vi "SmallestAngle.vi"(10 "Angle 2":dbl, 11 "Angle 1":dbl) -> (3 "Smallest Difference":dbl)   [LabVIEW 2016]
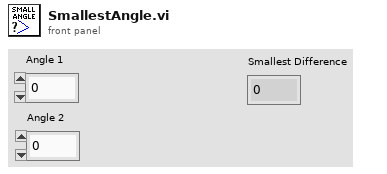
[diagram p1: front panel]
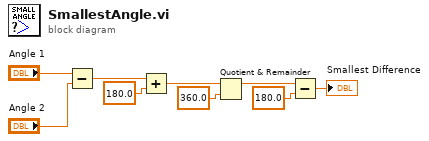
[diagram p0: block diagram]
diagram:
  n1 = Subtract(x="Angle 1", y="Angle 2") -> (x-y=w4:dbl)
  n2 = Add(x=w4, y=180.0) -> (x+y=w8:dbl)
  n3 = Quotient & Remainder(x=w8, y=360.0) -> (x-y*floor(x/y)=w6:dbl)  [unwired: 1 out]
  n4 = Subtract(x=w6, y=180.0 ("x-y*floor(x/y)")) -> (x-y=→"Smallest Difference":dbl)
